vi "initSound.vi"(0 "Error Message":string="Problemas al Inicializar el Sonido", 1 "Sound Parameters":T4) -> (2 "Sound Device OUT":T3 {"task ID" format="%.0x"}, 3 "# samples":u32, 4 "Inizializo?":bool, 5 "task ID":T1 format="%.0x")   [LabVIEW 2010]
uses:
  <vilib>/sound2/lvsound2.llb/Sound Data Format.ctl
  <vilib>/sound2/lvsound2.llb/Sound Output Task ID.ctl
  <vilib>/sound2/lvsound2.llb/Sampling Mode.ctl
  <vilib>/Utility/error.llb/DialogType.ctl
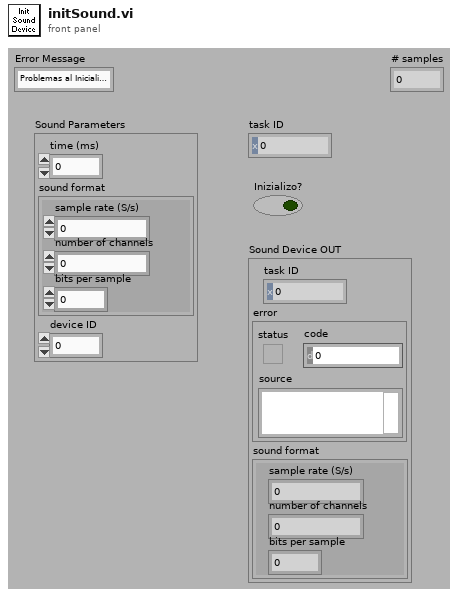
[diagram p1: front panel]
types:
  T1 = typedef "Sound Output Task ID.ctl" = u32
  T2 = typedef "Sound Data Format.ctl" = cluster{"sample rate (S/s)":dbl, "number of channels":i32, "bits per sample":i32}
  T3 = cluster{"task ID":T1, "error":errorcluster, "sound format":T2}
  T4 = cluster{"time (ms)":dbl, "sound format":T2, "device ID":u32}
  T5 = typedef "DialogType.ctl" = u16
  T6 = typedef "Sampling Mode.ctl" = i32
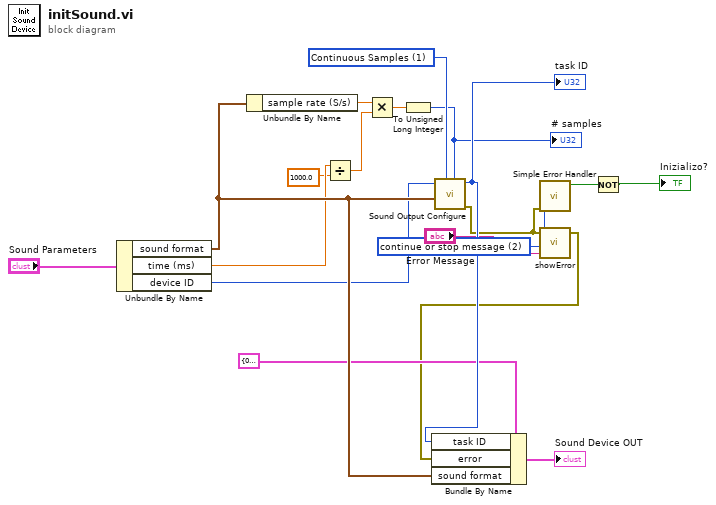
[diagram p0: block diagram]
diagram:
  w1 = T5 2 items=["no dialog", "OK message", "continue or stop message", "OK message + warnings", "continue/stop + warnings"] ("type of dialog (OK msg:1)")
  w12 = T6 1 items=["Finite Samples", "Continuous Samples"] ("sample mode")
  n1 = Unbundle By Name("Sound Parameters") -> ("sound format"=w18:T2, "time (ms)"=w14:dbl, "device ID"=w13:u32)
  n2 = Unbundle By Name(w18) -> ("sample rate (S/s)"=w9:dbl)
  n3 = Divide(x=w14, y=sgl 1000.0) -> (x/y=w8:dbl)
  n4 = Multiply(x=w9, y=w8) -> (x*y=w11:dbl)
  n5 = To Unsigned Long Integer(number=w11) -> (unsigned 32bit integer=w7:u32)
  "# samples" <- w7
  n6 = call <vilib>:"Sound Output Configure.vi"("number of samples/ch"=w7, "sample mode"=w12, "sound format"=w18, "device ID"=w13) -> ("error out"=w2:errorcluster, "task ID"=w17:T1)  [unwired: 6 in]
  "task ID" <- w17
  n7 = call <vilib>:"Simple Error Handler.vi"("type of dialog (OK msg:1)"=w1, "error in (no error)"=w2) -> ("error?"=w6:bool)  [unwired: 3 in, 4 out]
  n8 = call "showError.vi"("message"="Error Message", "Error IN"=w2) -> ("Error OUT"=w3:errorcluster)  [unwired: 3 in]
  n9 = Bundle By Name(cluster=T3 {"task ID"=0, "error"={"status"=FALSE, "code"=0, "source"=""}, "sound format"={"sample rate (S/s)"=0.0, "number of channels"=0, "bits per sample"=0}} ("Sound Device IN"), "task ID"=w17, "error"=w3, "sound format"=w18) -> (→"Sound Device OUT":T3)
  n10 = Not(x=w6) -> (.not. x?=→"Inizializo?":bool)
